vi "PrepareDataForPlot.vi"(5 "Sample Rate":dbl, 6 "Start Time (ms)":u32, 7 "Buffer Length":i32, 9 "Graph Buffer In":dbl[][](array[numeric]), 11 "New Samples":dbl[](array[numeric])) -> (1 "Graph Buffer Out":dbl[][](array[numeric]), 2 "WaveForm Data":cluster{dbl, dbl, dbl[][]})   [LabVIEW 2013]
doc: "This VI updates an array (<B>Graph Buffer</B>) with new data and creates a waveform object (<B>Waveform Data</B>) with data which can be used for plotting. Each column contains a time series of data and each row contains a timepoint for each time series.\n\nParameters:\n Start Time - Time in ms when data acquisition started\n Sampling Rate - Sampling rate of data acquisition\n New Samples - New samples to add to buffer (Consider doing that in separate VI)\n Buffer Length - Number of data elements in each time series."
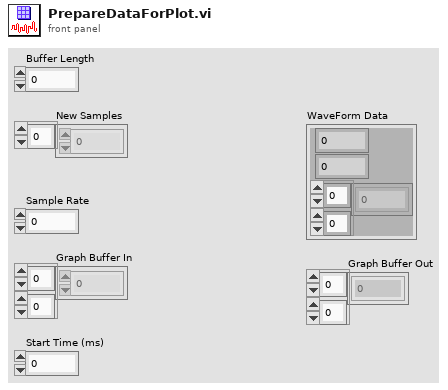
[diagram p1: front panel]
types:
  T1 = cluster{"Start time":dbl, "Delta t":dbl, "Time Series":dbl[][]}
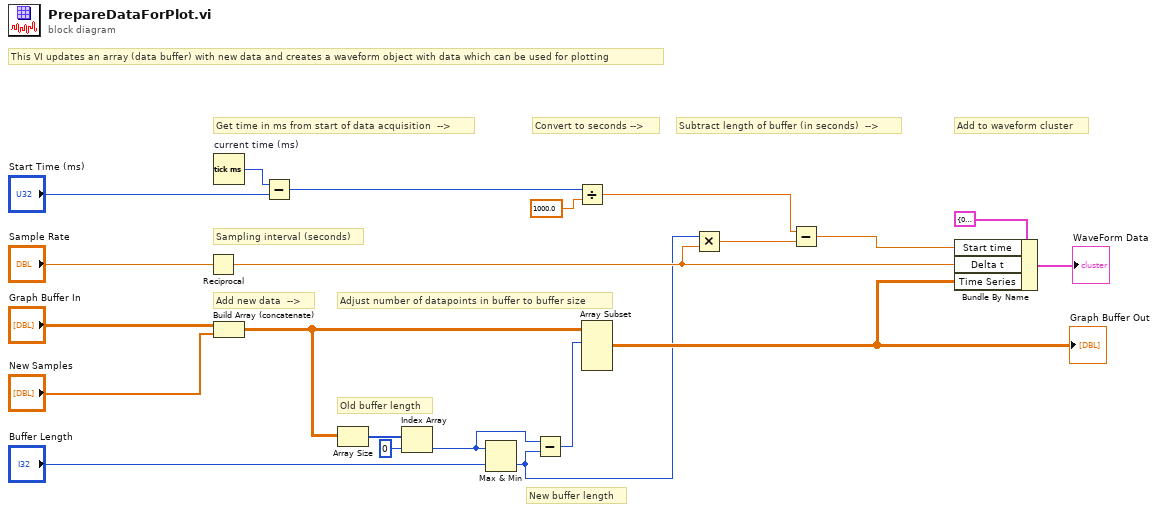
[diagram p0: block diagram]
diagram:
  # "Add to waveform cluster"
  # "Subtract length of buffer (in seconds)  -->"
  # "Convert to seconds -->"
  # "New buffer length"
  # "Old buffer length"
  # "Get time in ms from start of data acquisition  -->"
  # "Add new data  -->"
  # "Sampling interval (seconds)"
  # "This VI updates an array (data buffer) with new data and creates a waveform object with data which can be used for plotting"
  # "Adjust number of datapoints in buffer to buffer size"
  n1 = Reciprocal(x="Sample Rate") -> (1/x=w8:dbl)
  n2 = Tick Count (ms) "current time (ms)"() -> (millisecond timer value=w21:u32)
  n3 = Build Array (concatenate)("Graph Buffer In", "New Samples") -> (w12:dbl[][])
  n4 = Subtract(x=w21, y="Start Time (ms)") -> (x-y=w6:u32)
  n5 = Array Size(array=w12) -> (size(s)=w13:i32[])
  n6 = Index Array(array=w13, index=0) -> (element=w1:i32)
  n7 = Max & Min(x=w1, y="Buffer Length") -> (min(x,y)=w7:i32)  [unwired: 1 out]
  n8 = Subtract(x=w1, y=w7) -> (x-y=w16:i32)
  n9 = Divide(x=w6, y=1000.0) -> (x/y=w4:dbl)
  n10 = Array Subset(array=w12, index (row)=w16) -> (w19:dbl[][])  [unwired: 3 in]
  "Graph Buffer Out" <- w19
  n11 = Multiply(x=w7, y=w8) -> (x*y=w3:dbl)
  n12 = Subtract(x=w4, y=w3) -> (x-y=w5:dbl)
  n13 = Bundle By Name(cluster=T1 {"Start time"=0.0, "Delta t"=0.0, "Time Series"=[]}, "Start time"=w5, "Delta t"=w8, "Time Series"=w19) -> (→"WaveForm Data":T1)
